vi "04 - Demonstration - Effect of Branching Event Registration.vi"() -> ()   [LabVIEW 2012]
panel:
  out "Total Events Handled (chart)":i32(graph)
  out "Sum of Events Handled":i32
  out "Total Events Handled":i32
  out "Chart 3":i32(graph)
  out "Chart 2":i32(graph)
  in  "Event Registration Type?":enum16{"Unique (good!)", "Shared (bad!)"}(ring)
  out "Chart 1":i32(graph)
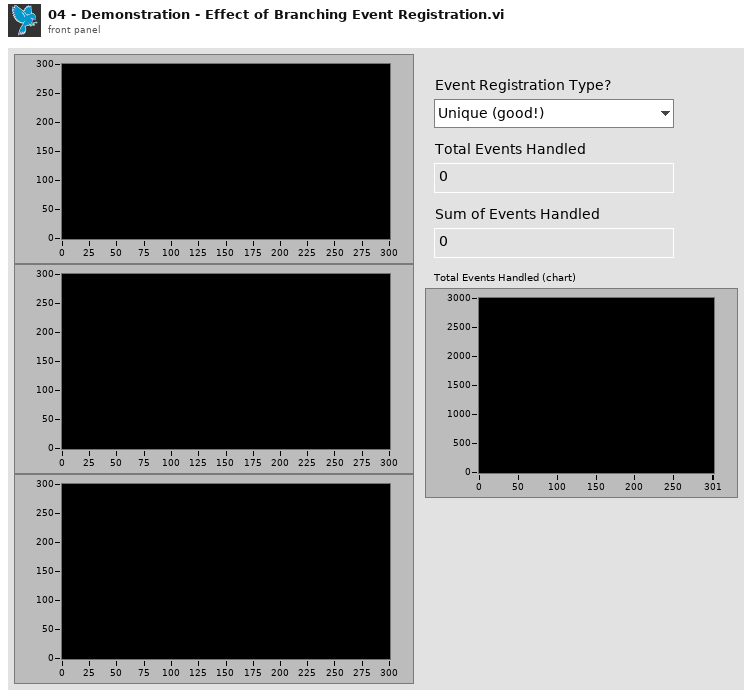
[diagram p1: front panel]
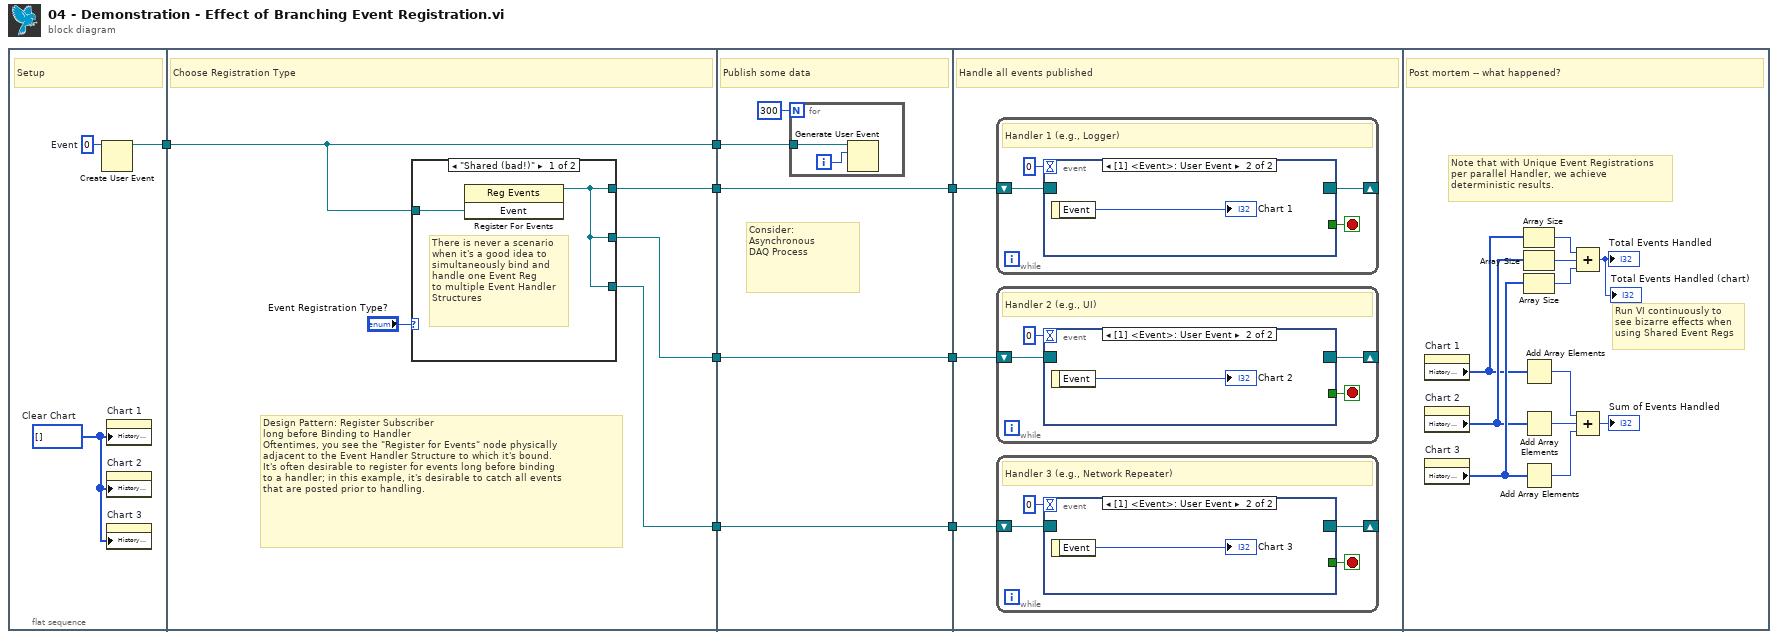
[diagram p0: block diagram]
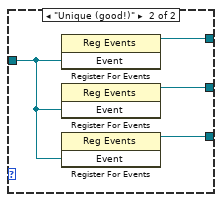
[diagram p2: hidden frame]
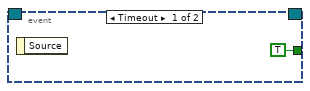
[diagram p3: hidden frame]
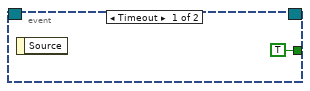
[diagram p4: hidden frame]
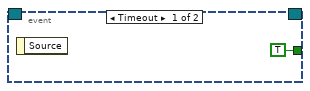
[diagram p5: hidden frame]
diagram:
  n1 = flat-sequence {
    tunnel: [w9] -> w1
    tunnel: [w16] -> w5
    tunnel: [w14] -> w4
    tunnel: [w13] -> w3
    tunnel: [w12] -> w2
    tunnel: w1 -> [w12]
    tunnel: [w27] -> w8
    tunnel: [w26] -> w7
    tunnel: [w25] -> w6
    tunnel: w5 -> [w27]
    tunnel: w4 -> [w26]
    tunnel: w3 -> [w25]
    tunnel: w2 -> [w23]
    tunnel: w8 -> [w32]
    tunnel: w7 -> [w31]
    tunnel: w6 -> [w30]
    frame #0 {
      w10 = 0  # Event
      w11 = i32[] []  # Clear Chart
      # "Setup"
      n2 = Create User Event(user event datatype=w10) -> (user event=w9:refnum<user-event>)  [unwired: 1 in, 1 out]
      n3 = property on="Chart 1" class="WFChart (strict)"("History Data"=w11) -> ()  [unwired: 2 in, 2 out]
      n4 = property on="Chart 2" class="WFChart (strict)"("History Data"=w11) -> ()  [unwired: 2 in, 2 out]
      n5 = property on="Chart 3" class="WFChart (strict)"("History Data"=w11) -> ()  [unwired: 2 in, 2 out]
    }
    frame #1 {
      # "Design Pattern: Register Subscriber\nlong before Binding to Handler\nOftentimes, you see the \"Register for Events\" node physically\nadjacent to the Event Handler Structure to which it's bound.\nIt's often desirable to register for events long before binding\nto a handler; in this example, it's desirable to catch all events\nthat are posted prior to handling."
      # "Choose Registration Type"
      n6 = case shown="\"Shared (bad!)\"" "Event Registration Type?" {
        tunnel: w12 -> [w18 w19]
        tunnel: [w17 w22] -> w16
        tunnel: [w17 w20] -> w14
        tunnel: [w17 w21] -> w13
        frame "Shared (bad!)" {
          # "There is never a scenario\nwhen it's a good idea to\nsimultaneously bind and\nhandle one Event Reg\nto multiple Event Handler\nStructures"
          n7 = register-events(w18) -> (reference out=w17:refnum<event-registration>)  [unwired: 2 in, 1 out]
        }
        frame "Unique (good!)" {
          n8 = register-events(w19) -> (reference out=w22:refnum<event-registration>)  [unwired: 2 in, 1 out]
          n9 = register-events(w19) -> (reference out=w20:refnum<event-registration>)  [unwired: 2 in, 1 out]
          n10 = register-events(w19) -> (reference out=w21:refnum<event-registration>)  [unwired: 2 in, 1 out]
        }
      }
    }
    frame #2 {
      # "Consider:\nAsynchronous\nDAQ Process"
      # "Publish some data"
      n11 = for {
        N: 300 -> [_]
        tunnel: w23 -> [w29]
        i -> [w28]
        n12 = Generate User Event(user event=w29, event data cluster=w28) -> ()  [unwired: 1 in, 2 out]
      }
    }
    frame #3 {
      # "Handle all events published"
      n13 = while {
        shift-right: [w47] -> _
        shift-left: w32 -> [w48]
        stop <- w46 stop-if-true
        # "Handler 1 (e.g., Logger)"
        n14 = event shown="[1] <Event>: User Event" {
          selector: w48 -> [_ _]
          dyn-events: [_ _] -> w47
          timeout: 0 -> [_ _]
          tunnel: [TRUE _] -> w46
          event Timeout {
            n15 = event-data() -> ()  [unwired: 1 in, 1 out]
          }
          event User Event {
            n16 = event-data() -> ("Event"=→"Chart 1":i32)  [unwired: 1 in]
          }
        }
      }
      n17 = while {
        shift-right: [w41] -> _
        shift-left: w31 -> [w42]
        stop <- w40 stop-if-true
        # "Handler 2 (e.g., UI)"
        n18 = event shown="[1] <Event>: User Event" {
          selector: w42 -> [_ _]
          dyn-events: [_ _] -> w41
          timeout: 0 -> [_ _]
          tunnel: [TRUE _] -> w40
          event Timeout {
            n19 = event-data() -> ()  [unwired: 1 in, 1 out]
          }
          event User Event {
            n20 = event-data() -> ("Event"=→"Chart 2":i32)  [unwired: 1 in]
          }
        }
      }
      n21 = while {
        shift-right: [w35] -> _
        shift-left: w30 -> [w36]
        stop <- w34 stop-if-true
        # "Handler 3 (e.g., Network Repeater)"
        n22 = event shown="[1] <Event>: User Event" {
          selector: w36 -> [_ _]
          dyn-events: [_ _] -> w35
          timeout: 0 -> [_ _]
          tunnel: [TRUE _] -> w34
          event Timeout {
            n23 = event-data() -> ()  [unwired: 1 in, 1 out]
          }
          event User Event {
            n24 = event-data() -> ("Event"=→"Chart 3":i32)  [unwired: 1 in]
          }
        }
      }
    }
    frame #4 {
      # "Run VI continuously to\nsee bizarre effects when\nusing Shared Event Regs"
      # "Note that with Unique Event Registrations\nper parallel Handler, we achieve\ndeterministic results."
      # "Post mortem -- what happened?"
      n25 = property on="Chart 1" class="WFChart (strict)"() -> ("History Data"=w59:i32[])  [unwired: 2 in, 2 out]
      n26 = property on="Chart 2" class="WFChart (strict)"() -> ("History Data"=w60:i32[])  [unwired: 2 in, 2 out]
      n27 = property on="Chart 3" class="WFChart (strict)"() -> ("History Data"=w61:i32[])  [unwired: 2 in, 2 out]
      n28 = Array Size(array=w59) -> (size(s)=w58:i32)
      n29 = Array Size(array=w60) -> (size(s)=w57:i32)
      n30 = Array Size(array=w61) -> (size(s)=w56:i32)
      n31 = Add Array Elements(numeric array=w59) -> (sum=w54:i32)
      n32 = Add Array Elements(numeric array=w60) -> (sum=w55:i32)
      n33 = Add Array Elements(numeric array=w61) -> (sum=w53:i32)
      n34 = Compound Arithmetic op=ADD(w58, w57, w56) -> (→"Total Events Handled" →"Total Events Handled (chart)":i32)
      n35 = Compound Arithmetic op=ADD(w54, w55, w53) -> (→"Sum of Events Handled":i32)
    }
  }
